vi "Initialize Control Appearance.vi"(8 "error in (no error)":errorcluster, 11 "Selector in":refnum<class "Selector.lvclass">) -> (0 "error out":errorcluster, 3 "Selector out":refnum<class "Selector.lvclass">)   [LabVIEW 2019, in "Selector.lvclass"]
uses:
  Selector.lvclass
  <vilib>/Utility/miscctls.llb/LVRowAndColumnUnsignedTypeDef.ctl
  <vilib>/Utility/miscctls.llb/LVRowAndColumnTypeDef.ctl
  Selector.lvclass/Selector.ctl
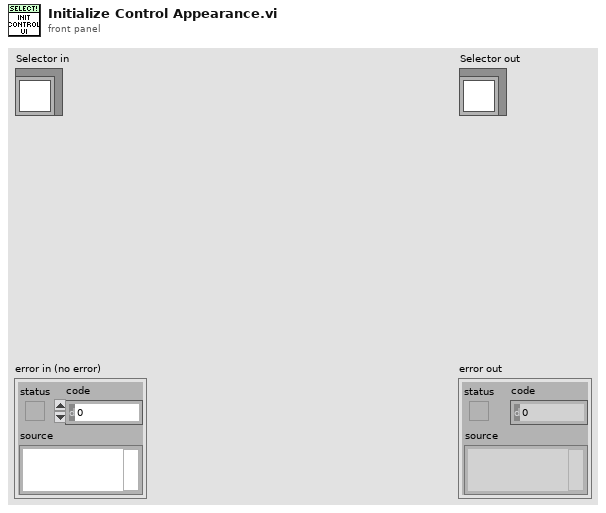
[diagram p1: front panel]
types:
  T1 = typedef "LVRowAndColumnTypeDef.ctl" = cluster{"Row":i32, "Column":i32}
  T2 = typedef "LVRowAndColumnUnsignedTypeDef.ctl" = cluster{"Row":u32, "Column":u32}
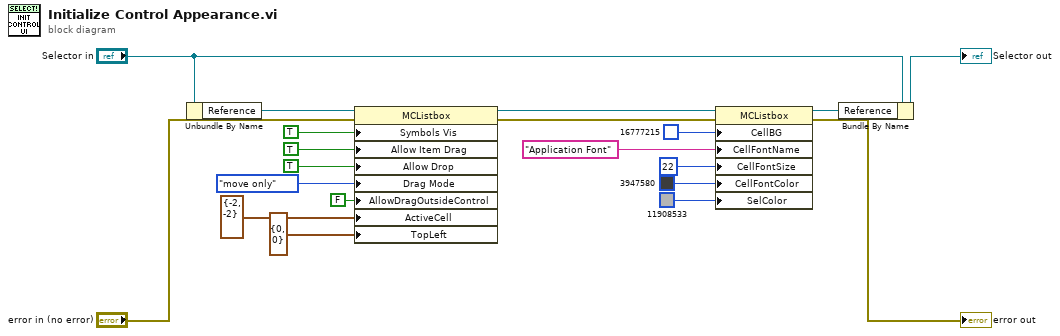
[diagram p0: block diagram]
diagram:
  n1 = Unbundle By Name("Selector in") -> ("Reference"=w20:refnum<vi>)
  n2 = property class="MCListbox"(reference=w20, error in="error in (no error)", "Symbols Vis"=TRUE ("Visible Items:Symbols Visible"), "Allow Item Drag"=TRUE ("Drag/Drop:Allow Dragging"), "Allow Drop"=TRUE ("Drag/Drop:Allow Dropping"), "Drag Mode"=enum32{"copy or move", "copy only", "move only"}."move only" ("Drag/Drop:Drag Mode"), "AllowDragOutsideControl"=FALSE ("Drag/Drop:Allow Drag and Drop Outside Control"), "ActiveCell"=T1 {"Row"=-2, "Column"=-2} ("Active Cell:Active Cell"), "TopLeft"=T2 {"Row"=0, "Column"=0} ("Top Left Visible Cell")) -> (reference out=w7:refnum<vi>, error out=w6:errorcluster)
  n3 = property class="MCListbox"(reference=w7, error in=w6, "CellBG"=u32 16777215 ("Active Row:Cell Background Color"), "CellFontName"="Application Font" ("Font Name"), "CellFontSize"=u32 22 ("Size"), "CellFontColor"=u32 3947580 ("Color"), "SelColor"=u32 11908533 ("Active Row:Cell Background Color")) -> (reference out=w5:refnum<vi>, error out=→"error out":errorcluster)
  n4 = Bundle By Name(cluster="Selector in", "Reference"=w5) -> (→"Selector out":refnum<class "Selector.lvclass">)
